vi "Set Phys Instr.vi"(10 "Phys Instr":T1(c390), 11 "MSS in":refnum<class "MSS.lvclass">) -> (3 "MSS out":refnum<class "MSS.lvclass">)   [LabVIEW 2023]
uses:
  MSS.lvclass
  HAL GOOP4/Instrument/Instrument.lvclass
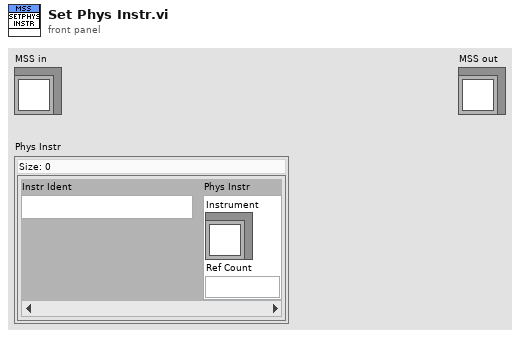
[diagram p1: front panel]
types:
  T1 = map{string, cluster{"Instrument":refnum<class "Instrument.lvclass">, "Ref Count":u8}}
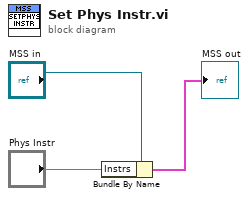
[diagram p0: block diagram]
diagram:
  n1 = Bundle By Name(cluster="MSS in", "Instrs"="Phys Instr") -> (→"MSS out":cluster{})
